vi "Global rpm nom.vi"() -> ()   [LabVIEW 2019]
panel:
  in  "rpm nom":dbl
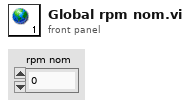
[diagram p1: front panel]
diagram:
